vi "Colorify.vi"(8 "Front Panel":refnum<vi>, 9 "String 2":refnum<vi>, 11 "String":string) -> ()   [LabVIEW 2020]
uses:
  ColorText/ColorGlobals.vi
panel:
  out "End":i32
  out "Start":i32
  out "Occurances":i32
  out "Line Number":i32
  out "Good?":bool
  out "Before Error":i32
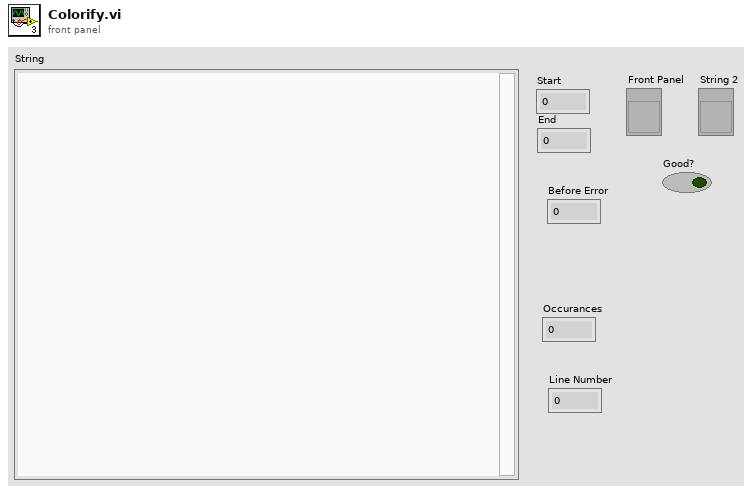
[diagram p1: front panel]
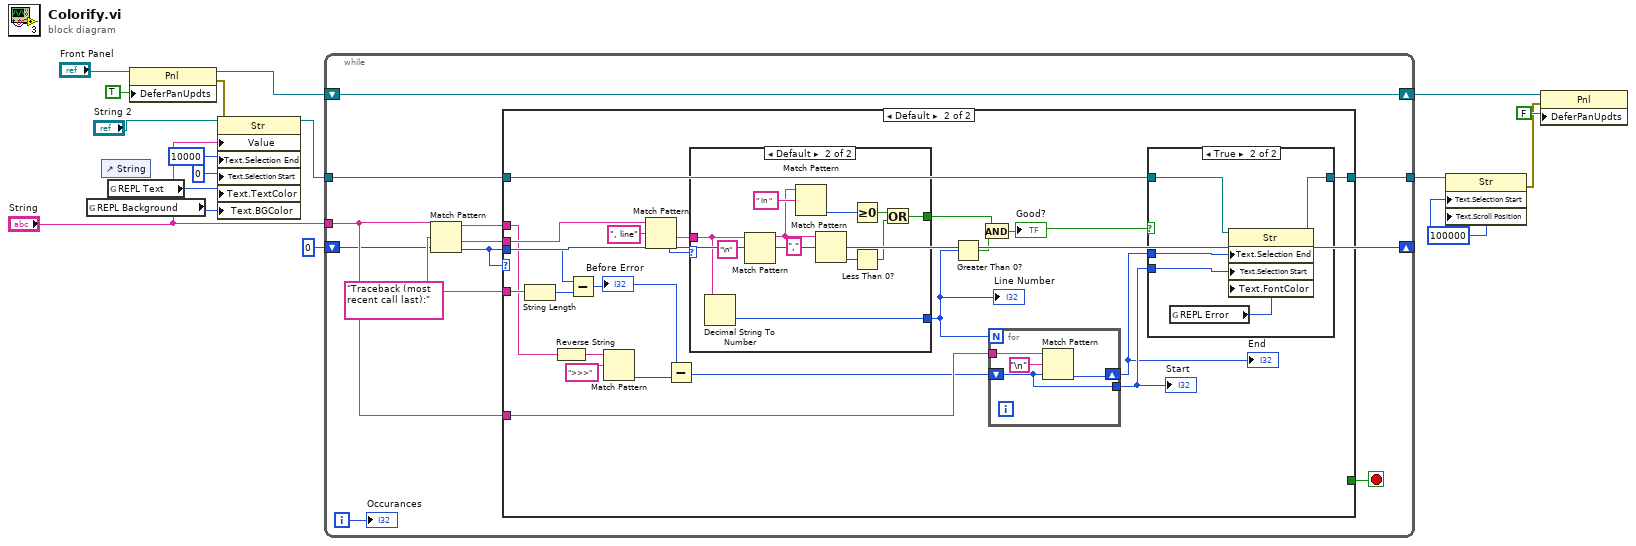
[diagram p0: block diagram]
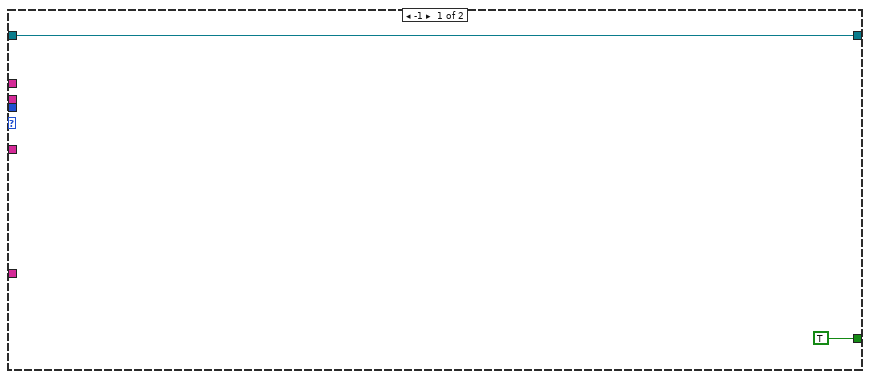
[diagram p2: hidden frame]
diagram:
  w8 = u32 100000 ("Text.Selection:Start")
  n1 = global read "ColorGlobals.vi" "REPL Background"() -> (w1:u32)
  n2 = control-ref of="String"() -> ()  [unwired: 1 out]
  n3 = global read "ColorGlobals.vi" "REPL Text"() -> (w2:u32)
  n4 = property class="Pnl"(reference="Front Panel", "DeferPanUpdts"=TRUE ("Defer Panel Updates")) -> (reference out=w14:refnum<vi>, error out=w3:errorcluster)  [unwired: 1 in]
  n5 = property on="Property Node" class="Str"(reference="String 2", error in=w3, "Value"="String", "Text.Selection End"=u32 10000 ("Text.Selection:End"), "Text.Selection Start"=u32 0 ("Text.Selection:Start"), "Text.TextColor"=w2, "Text.BGColor"=w1) -> (reference out=w6:refnum<vi>)  [unwired: 1 out]
  n6 = while {
    tunnel: "String" -> [w25]
    shift-right: [w23] -> w15
    shift-left: w14 -> [w23]
    shift-right: [w22] -> _
    shift-left: 0 ("offset (0)") -> [w24]
    tunnel: w6 -> [w20]
    tunnel: [w18] -> w5
    i -> [w19]
    stop <- w21 stop-if-true
    w28 = "Traceback (most recent call last):"
    n7 = Match Pattern(string=w25, regular expression=w28, offset (0)=w24) -> (before substring=w26:string, after substring=w27:string, offset past match=w22:i32)  [unwired: 1 out]
    n8 = case shown="Default" w22 {
      tunnel: w28 -> [_ w51]
      tunnel: w27 -> [_ w44]
      tunnel: w26 -> [_ w41]
      tunnel: w25 -> [_ w40]
      tunnel: w22 -> [_ w36]
      tunnel: [TRUE _] -> w21
      tunnel: w20 -> [w29 w34]
      tunnel: [w29 w31] -> w18
      frame -1 {
      }
      frame Default {
        n9 = String Length(string=w51) -> (length=w52:i32)
        n10 = Reverse String(1:w41) -> (0:w43:string)
        n11 = Subtract(x=w36, y=w52) -> (x-y=w35:i32)
        "Before Error" <- w35
        n12 = Match Pattern(string=w43, regular expression=">>>") -> (offset past match=w33:i32)  [unwired: 1 in, 3 out]
        n13 = Match Pattern(string=w44, regular expression=", line") -> (after substring=w49:string, offset past match=w46:i32)  [unwired: 1 in, 2 out]
        n14 = Subtract(x=w35, y=w33) -> (x-y=w32:i32)
        n15 = case shown="Default" w46 {
          tunnel: w49 -> [_ w65]
          tunnel: [_ w64] -> w47
          tunnel: [_ w63] -> w38
          frame -1 {
          }
          frame Default {
            n16 = Decimal String To Number(string=w65) -> (number=w63:i32)  [unwired: 2 in, 1 out]
            n17 = Match Pattern(string=w65, regular expression="\n") -> (before substring=w69:string)  [unwired: 1 in, 3 out]
            n18 = Match Pattern(string=w69, regular expression=" in ") -> (offset past match=w70:i32)  [unwired: 1 in, 3 out]
            n19 = Match Pattern(string=w69, regular expression=",") -> (offset past match=w68:i32)  [unwired: 1 in, 3 out]
            n20 = Greater Or Equal To 0?(x=w70) -> (x >= 0?=w66:bool)
            n21 = Less Than 0?(x=w68) -> (x < 0?=w67:bool)
            n22 = Or(x=w66, y=w67) -> (x .or. y?=w64:bool)
          }
        }
        "Line Number" <- w38
        n23 = Greater Than 0?(x=w38) -> (x > 0?=w48:bool)
        n24 = And(x=w47, y=w48) -> (x .and. y?=w45:bool)
        "Good?" <- w45
        n25 = for {
          N: w38 -> [_]
          tunnel: w40 -> [w56]
          shift-right: [w54] -> w37
          shift-left: w32 -> [w53]
          tunnel: [w53] -> w39
          n26 = Match Pattern(string=w56, regular expression="\n", offset (0)=w53) -> (offset past match=w54:i32)  [unwired: 3 out]
        }
        "Start" <- w39
        "End" <- w37
        n27 = case shown="True" w45 {
          tunnel: w37 -> [_ w59]
          tunnel: w39 -> [_ w60]
          tunnel: w34 -> [w57 w62]
          tunnel: [w57 w61] -> w31
          frame False {
          }
          frame True {
            n28 = global read "ColorGlobals.vi" "REPL Error"() -> (w58:u32)
            n29 = property on="Property Node" class="Str"(reference=w62, "Text.Selection End"=w59, "Text.Selection Start"=w60, "Text.FontColor"=w58) -> (reference out=w61:refnum<vi>)  [unwired: 1 in, 1 out]
          }
        }
      }
    }
    "Occurances" <- w19
  }
  n30 = property on="Property Node" class="Str"(reference=w5, "Text.Selection Start"=w8, "Text.Scroll Position"=w8) -> (error out=w7:errorcluster)  [unwired: 1 in, 1 out]
  n31 = property class="Pnl"(reference=w15, error in=w7, "DeferPanUpdts"=FALSE ("Defer Panel Updates")) -> ()  [unwired: 2 out]
